vi "GS Range.vi"() -> ()   [LabVIEW 2020, in "Yokogawa GX Series.lvlib"]
uses:
  <instrlib>/Yokogawa GX Series/Yokogawa GX Series.lvlib
panel:
  in  "GS Range":string="1-5V\n0.4-2V"
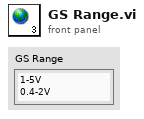
[diagram p1: front panel]
diagram:
